vi "Write StimulationPath.vi"(8 "error in (no error)":errorcluster, 10 "StimulationPath":path, 11 "MatlabExperiment in":refnum<class "MatlabExperiment.lvclass">) -> (0 "error out":errorcluster, 3 "MatlabExperiment out":refnum<class "MatlabExperiment.lvclass">)   [LabVIEW 2014, in "AcquisitionCoreObjects.lvlib" / "MatlabExperiment.lvclass"]
uses:
  MatlabExperiment.lvclass
  MatlabExperiment.lvclass/MatlabExperiment.ctl
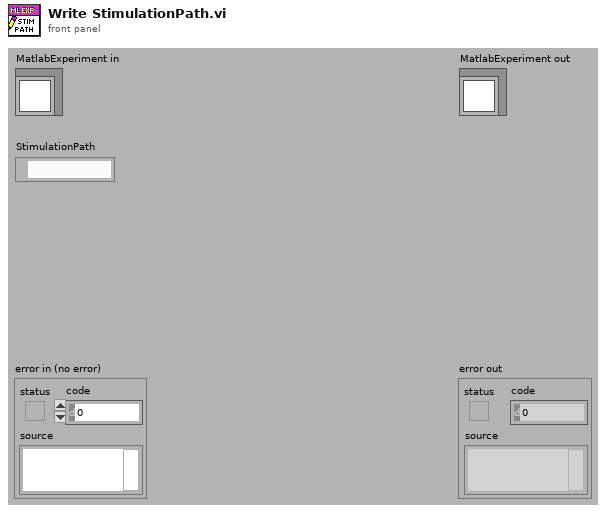
[diagram p1: front panel]
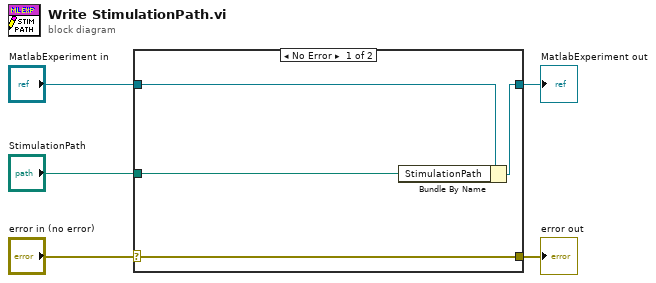
[diagram p0: block diagram]
diagram:
  n1 = case shown="No Error" "error in (no error)" {
    selector: "error in (no error)" -> [w9 w10]
    tunnel: [w9 w10] -> w4
    tunnel: [w7 w11] -> w2
    tunnel: "MatlabExperiment in" -> [w8 w11]
    tunnel: "StimulationPath" -> [w6 _]
    frame No Error {
      n2 = Bundle By Name(cluster=w8, "StimulationPath"=w6) -> (w7:refnum<class "MatlabExperiment.lvclass">)
    }
    frame Error {
    }
  }
  "error out" <- w4
  "MatlabExperiment out" <- w2
